vi "light sensor.vi"   [LabVIEW 2012, in "sumobot 18.lvrbt"]
uses:
  sumobot 18.lvrbt
  <vilib>/NXT/Block Support/NXT_InputPort.ctl
  <vilib>/NXT/Block Support/NXT_OutputPort.ctl
  <vilib>/NXT/Dual Mode Library/Waits/Wait_Num.vi
  <vilib>/NXT/Dual Mode Library/Sensors/Light_On.vi
  <vilib>/NXT/NXTIO Xnodes/NXTIONodeSubVIs/NXTMoveMotors.vi
  <vilib>/NXT/NXTIO Xnodes/NXTIONodeSubVIs/LEGOStopAllMotors.vi
  <vilib>/NXT/NXTIO Xnodes/AddressXNode/NXTIOAddress.xnode
  <vilib>/NXT/NXTIO Xnodes/NXTIOXNode/NXTIO.xnode
  <vilib>/NXT/Subs/LVHSConnector.ctl
  <vilib>/NXT/LegoClasses/BrickReference/BrickReference.lvclass
types:
  T1 = typedef "LVHSConnector.ctl" = refnum<class "BrickReference.lvclass">
  T2 = typedef "NXT_OutputPort.ctl" = u8
  T3 = cluster{"Output Port":T2, "Output Port 2":T2, "Output Port 3":T2}
  T4 = typedef "NXT_InputPort.ctl" = u32
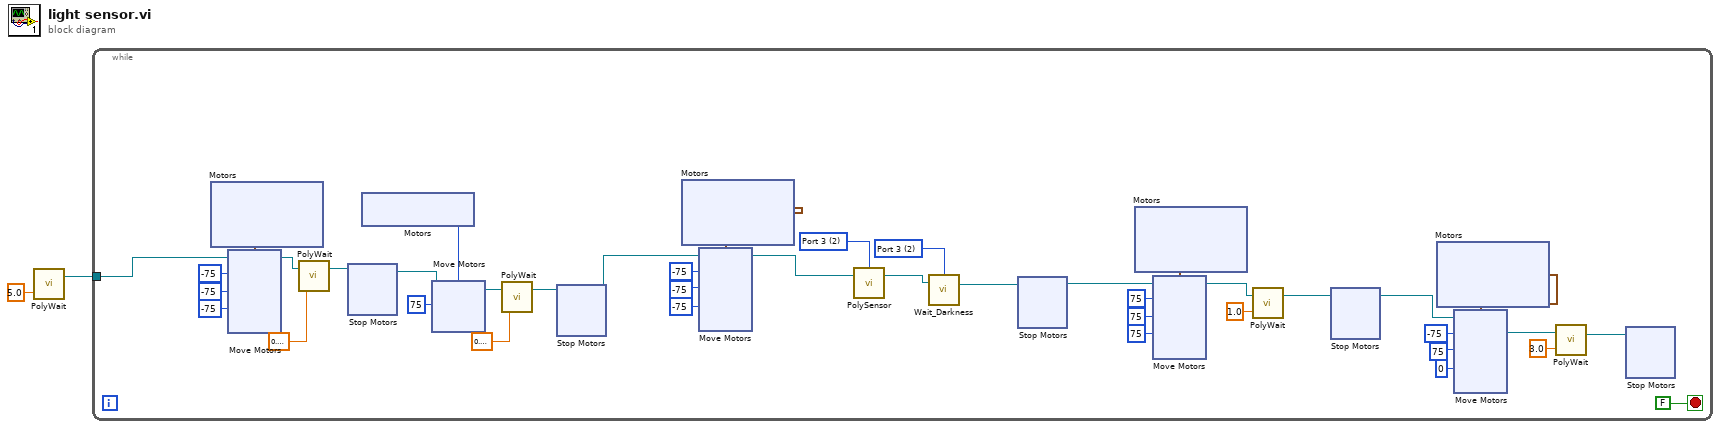
[diagram p0: block diagram]
diagram:
  n1 = call-poly <vilib>:"PolyWait.vi"("Time (1 sec)"=sgl 5.0) -> ("NXT/EV3"=w1:T1)  [unwired: 3 in]
  n2 = while {
    tunnel: w1 -> [w3]
    stop <- FALSE stop-if-true
    w41 = T4 2 items=["Port 1", "Port 2", "Port 3", "Port 4"] ("Port (Port 3)")
    w43 = T4 2 items=["Port 1", "Port 2", "Port 3", "Port 4"] ("Port (Port 3)")
    n3 = xnode "Motors"() -> ("Motor"=w40:cluster{"Port":T2, "Port":T2, "Port":T2})
    n4 = xnode "Move Motors"("Power/Speed 3"=i8 -75, "Power/Speed 2"=i8 -75, "Power/Speed 1"=i8 -75, "Motors"=w40, "NXT/EV3"=w3) -> ("NXT/EV3"=w25:T1)
    n5 = call-poly <vilib>:"PolyWait.vi"("Time (1 sec)"=sgl 0.3, "NXT/EV3"=w25) -> ("NXT/EV3"=w23:T1)  [unwired: 2 in]
    n6 = xnode "Stop Motors"("NXT/EV3"=w23) -> ("NXT/EV3"=w22:T1)  [unwired: 1 in]
    n7 = xnode "Motors"() -> ("Motor"=w27:T2)
    n8 = xnode "Move Motors"("Power/Speed 1"=i8 75, "Motors"=w27, "NXT/EV3"=w22) -> ("NXT/EV3"=w21:T1)
    n9 = call-poly <vilib>:"PolyWait.vi"("Time (1 sec)"=sgl 0.2, "NXT/EV3"=w21) -> ("NXT/EV3"=w19:T1)  [unwired: 2 in]
    n10 = xnode "Stop Motors"("NXT/EV3"=w19) -> ("NXT/EV3"=w13:T1)  [unwired: 1 in]
    n11 = xnode "Motors"() -> ("Motor"=w16:cluster{"Port":T2, "Port":T2, "Port":T2})
    n12 = xnode "Move Motors"("Power/Speed 3"=i8 -75, "Power/Speed 2"=i8 -75, "Power/Speed 1"=i8 -75, "Motors"=w16, "NXT/EV3"=w13) -> ("NXT/EV3"=w14:T1)
    n13 = call-poly <vilib>:"PolySensor.vi"("NXT/EV3"=w14, "Port (Port 3)"=w43) -> ("NXT/EV3"=w42:T1)  [unwired: 1 in, 1 out]
    n14 = call <vilib>:"Wait_Darkness.vi"("NXT/EV3"=w42, "Port (Port 3)"=w41) -> ("NXT/EV3"=w36:T1)  [unwired: 2 in]
    n15 = xnode "Stop Motors"("NXT/EV3"=w36) -> ("NXT/EV3"=w31:T1)  [unwired: 1 in]
    n16 = xnode "Motors"() -> ("Motor"=w35:cluster{"Port":T2, "Port":T2, "Port":T2})
    n17 = xnode "Move Motors"("Power/Speed 1"=i8 75, "Motors"=w35, "NXT/EV3"=w31, "Power/Speed 3"=i8 75, "Power/Speed 2"=i8 75) -> ("NXT/EV3"=w30:T1)
    n18 = call-poly <vilib>:"PolyWait.vi"("Time (1 sec)"=sgl 1.0, "NXT/EV3"=w30) -> ("NXT/EV3"=w28:T1)  [unwired: 2 in]
    n19 = xnode "Stop Motors"("NXT/EV3"=w28) -> ("NXT/EV3"=w8:T1)  [unwired: 1 in]
    n20 = xnode "Motors"() -> ("Motor"=w10:cluster{"Port":T2, "Port":T2, "Port":T2})
    n21 = xnode "Move Motors"("Power/Speed 3"=i8 0, "Power/Speed 2"=i8 75, "Power/Speed 1"=i8 -75, "Motors"=w10, "NXT/EV3"=w8) -> ("NXT/EV3"=w7:T1)
    n22 = call-poly <vilib>:"PolyWait.vi"("Time (1 sec)"=sgl 3.0, "NXT/EV3"=w7) -> ("NXT/EV3"=w5:T1)  [unwired: 2 in]
    n23 = xnode "Stop Motors"("NXT/EV3"=w5) -> ()  [unwired: 1 in, 1 out]
  }
